vi "Crop (Greyscale).vi"(7 "Origin (Default: 0,0)":T1, 8 "error in (no error)":errorcluster, 9 "Cropped Size":T2, 10 "Greyscale Image Destination":T3, 11 "Greyscale Image Source":T3) -> (0 "error out":errorcluster, 3 "Greyscale Image Destination (duplicate)":T3)   [LabVIEW 2020, in "image.lvlib"]
uses:
  image.lvlib
  Greyscale Image.ctl
  common/Image Size (Integer).ctl
  common/Image Point (Integer).ctl
  2dc01dea-48f6-4df4-8727-934e95e7e307.vi
  common/Module Path.vi
  <vilib>/Utility/error.llb/Error Cluster From Error Code.vi
  common/common.lvlib
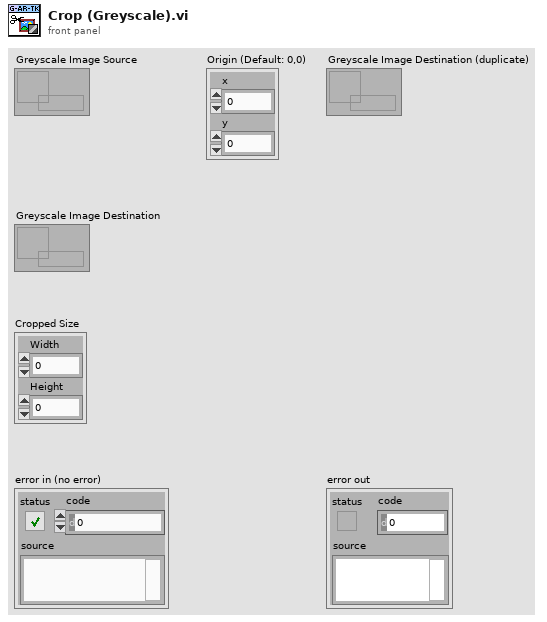
[diagram p1: front panel]
types:
  T1 = typedef "common.lvlib/Image Point (Integer).ctl" = cluster{"x":i32, "y":i32}
  T2 = typedef "common.lvlib/Image Size (Integer).ctl" = cluster{"Width":u16, "Height":u16}
  T3 = typedef "image.lvlib/Greyscale Image.ctl" = refnum<data-value>
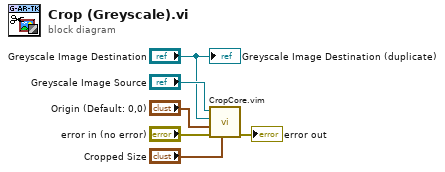
[diagram p0: block diagram]
diagram:
  n1 = call "CropCore.vim"("Size"="Cropped Size", "error in (no error)"="error in (no error)", "Origin"="Origin (Default: 0,0)", "Dst"="Greyscale Image Destination", "Src"="Greyscale Image Source") -> ("error out"=→"error out":errorcluster)  [unwired: 6 in]
  "Greyscale Image Destination (duplicate)" <- "Greyscale Image Destination"
